vi "Read Text Font.vi"(8 "error in (no error)":errorcluster, 11 "Control in":refnum<class "Control.lvclass">) -> (0 "error out":errorcluster, 2 "Font":T1={"Font Name:"="", "Size"=12, "Strikeout?"=FALSE, "Italic?"=FALSE, "Underline?"=FALSE, "Outline?"=FALSE, "Shadow?"=FALSE, "Bold?"=FALSE}, 3 "Control out":refnum<class "Control.lvclass">)   [LabVIEW 2012, in "Control.lvclass"]
uses:
  Control.lvclass
  Controls/_ui_tools_font.ctl
  Control.lvclass/Control.ctl
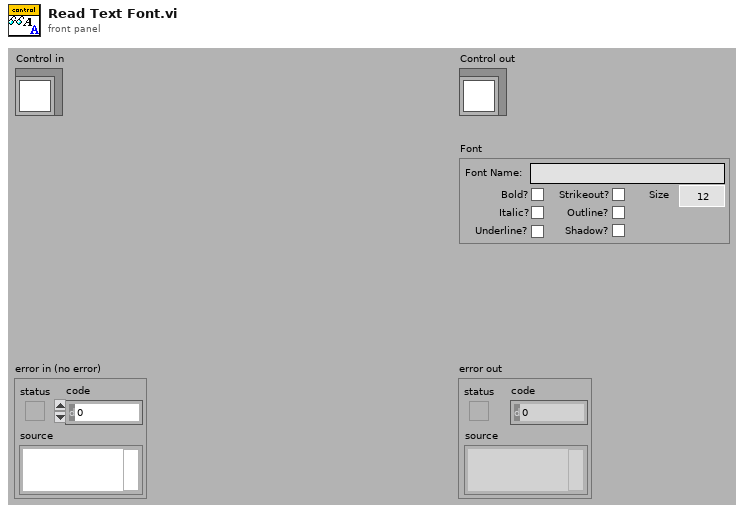
[diagram p1: front panel]
types:
  T1 = typedef "Control.lvclass/_ui_tools_font.ctl" = cluster{"Font Name:":string, "Size":i16, "Strikeout?":bool, "Italic?":bool, "Underline?":bool, "Outline?":bool, "Shadow?":bool, "Bold?":bool}
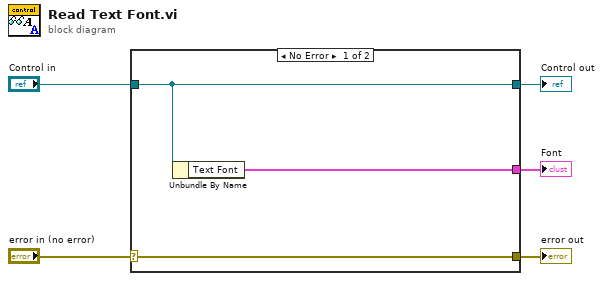
[diagram p0: block diagram]
diagram:
  n1 = case shown="No Error" "error in (no error)" {
    selector: "error in (no error)" -> [w8 w9]
    tunnel: [w8 w9] -> w4
    tunnel: [w7 w10] -> w2
    tunnel: "Control in" -> [w7 w10]
    tunnel: [w6 _] -> w1
    frame No Error {
      n2 = Unbundle By Name(w7) -> ("Text Font"=w6:T1)
    }
    frame Error {
    }
  }
  "error out" <- w4
  "Control out" <- w2
  "Font" <- w1
